vi "GetPosRef.vi"(0 "Entrée Variables d'Axes":T1={"OrdreBloc"="ni.var.psp://localhost/OPC/OPC1/esbimETH_1/module1/2AXBOC/E0_Ordre/Axe1_OrdreBloc", "Ordre UC"="ni.var.psp://localhost/OPC/OPC1/esbimETH_1/module1/2AXBOC/E0_Ordre/Axe1_OrdreUC", "CoteAAtteindre"="ni.var.psp://localhost/OPC/OPC1/esbimETH_1/module1/2AXBOC/E1_Position1/CoteAAtteindre", "Vitesse"="ni.var.psp://localhost/OPC/OPC1/esbimETH_1/module1/2AXBOC/E1_Position1/Vitesse", "Position codeur en pas"="ni.var.psp://localhost/OPC/OPC1/esbimETH_1/module1/2AXBOC/L4_PositionPas/Axe1_PositionCodeurEnPas", "Position Théorique"="ni.var.psp://localhost/OPC/OPC1/esbimETH_1/module1/2AXBOC/L0_Position/Axe1_PositionTheorique", "Message"="ni.var.psp://localhost/OPC/OPC1/esbimETH_1/module1/2AXBOC/L0_Position/Axe1_Messages", "Ecrire"="ni.var.psp://localhost/OPC/OPC1/esbimETH_1/module1/2AXBOC/ecrire", "Zone à écrire"="ni.var.psp://localhost/OPC/OPC1/esbimETH_1/module1/2AXBOC/zones_a_ecrire", "Numéro paramètre"="ni.var.psp://localhost/OPC/OPC1/esbimETH_1/module1/2AXBOC/E3_Parametres/NumeroParametre", "Ordre"="ni.var.psp://localhost/OPC/OPC1/esbimETH_1/module1/2AXBOC/E3_Parametres/Ordre", "Valeur"="ni.var.psp://localhost/OPC/OPC1/esbimETH_1/module1/2AXBOC/E3_Parametres/Valeur", "Valeur Lecture"="ni.var.psp://localhost/OPC/OPC1/esbimETH_1/module1/2AXBOC/L2_Parametres/Valeur", "Numéro paramètre Lecture"="ni.var.psp://localhost/OPC/OPC1/esbimETH_1/module1/2AXBOC/L2_Parametres/Numero", "Acquittement Lecture Ecriture"="", "Zone à Ecrire Pour Axe "=0, "Acquittement Ordre UC"=""}, 3 "error in (no error)":errorcluster caption="entrée d'erreur (pas d'erreur)") -> (9 "Références":i32[](array[numeric]), 10 "error out":errorcluster caption="sortie d'erreur")   [LabVIEW 2013]
uses:
  Controls/AdressesVariablesPartagees.ctl
  <vilib>/regexp/Match Regular Expression.xnode
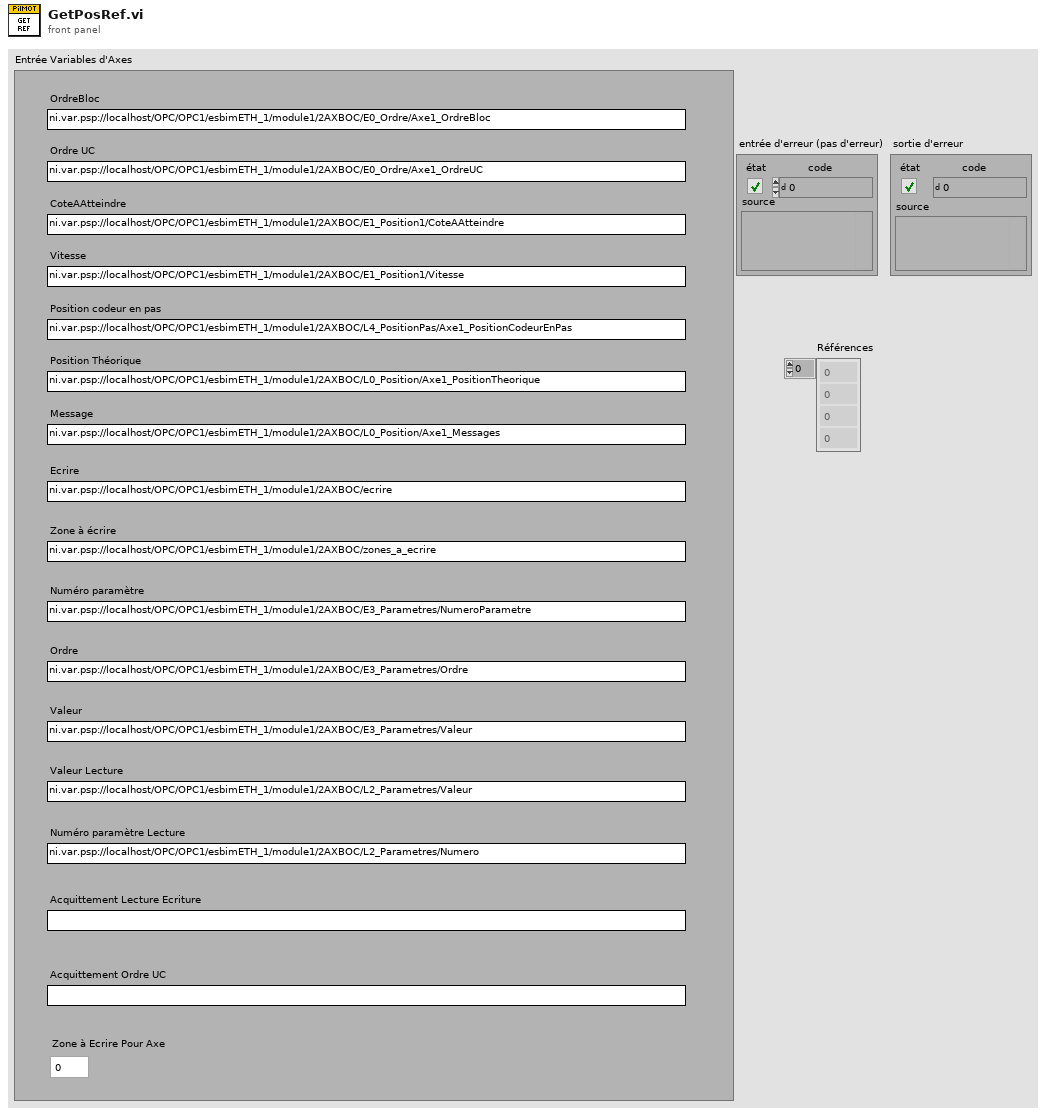
[diagram p1: front panel]
types:
  T1 = typedef "AdressesVariablesPartagees.ctl" = cluster{"OrdreBloc":string, "Ordre UC":string, "CoteAAtteindre":string, "Vitesse":string, "Position codeur en pas":string, "Position Théorique":string, "Message":string, "Ecrire":string, "Zone à écrire":string, "Numéro paramètre":string, "Ordre":string, "Valeur":string, "Valeur Lecture":string, "Numéro paramètre Lecture":string, "Acquittement Lecture Ecriture":string, "Zone à Ecrire Pour Axe ":u16, "Acquittement Ordre UC":string}
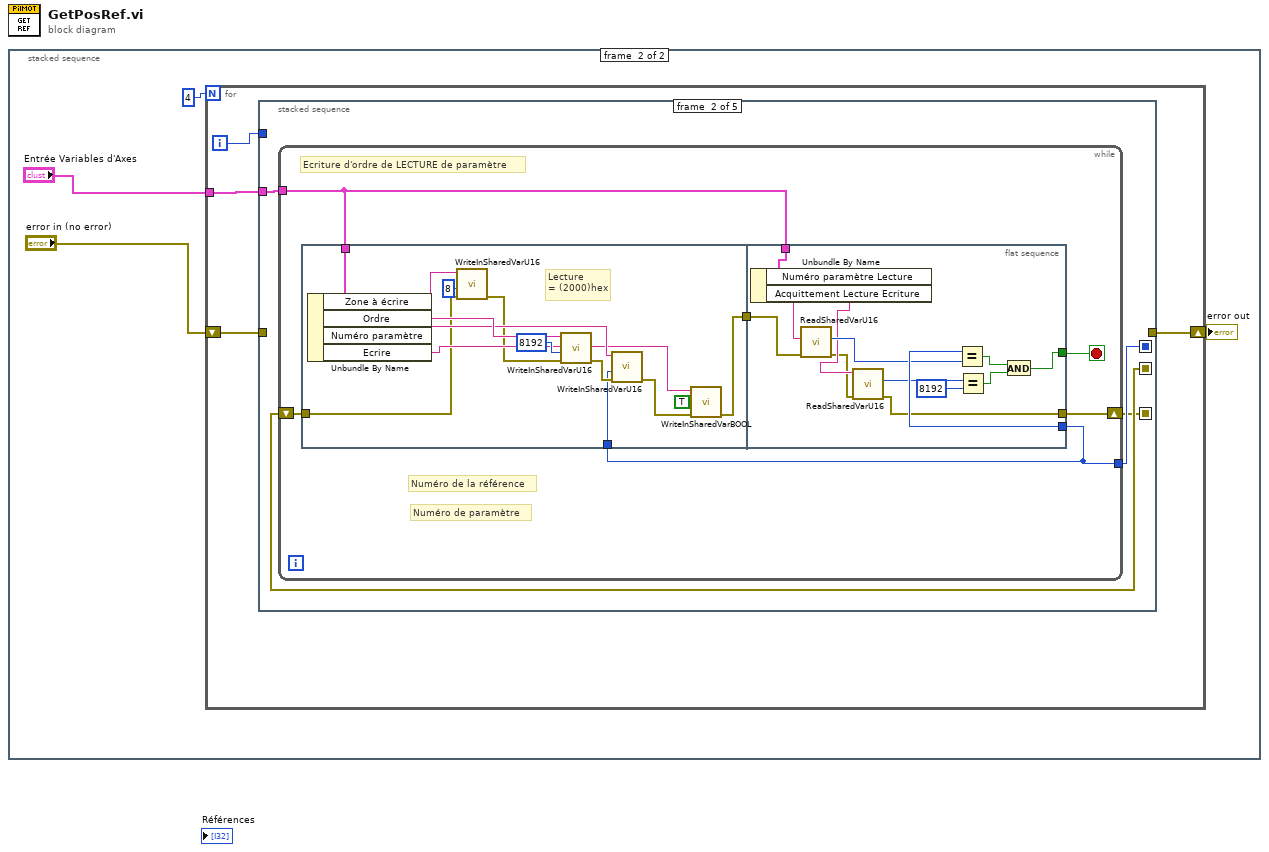
[diagram p0: block diagram]
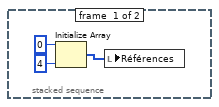
[diagram p2: hidden frame]
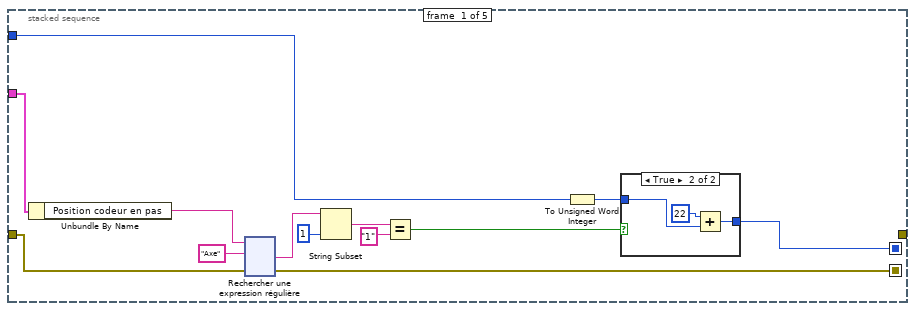
[diagram p3: hidden frame]
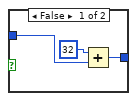
[diagram p4: hidden frame]
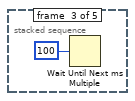
[diagram p5: hidden frame]
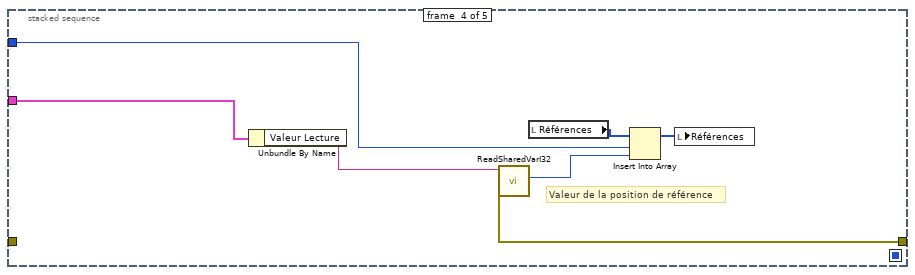
[diagram p6: hidden frame]
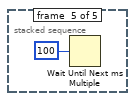
[diagram p7: hidden frame]
diagram:
  n1 = stacked-sequence {
    frame #0 {
      n2 = Initialize Array(0 ("élément"), 4 ("taille de la dimension")) -> (w1:i32[])
      n3 = local write "Références"(w1) -> ()
    }
    frame #1 {
      n4 = for {
        N: 4 -> [_]
        tunnel: "Entrée Variables d'Axes" -> [w11]
        shift-right: [w8] -> w5
        shift-left: "error in (no error)" -> [w9]
        i -> [w10]
        n5 = stacked-sequence {
          seq-local: [w16 _ _ _ _] -> [_ w146 _ _ _]
          seq-local: [w15 _ _ _ _] -> [_ w147 _ _ _]
          seq-local: [_ w145 _ _ _] -> [_ _ _ _ _]
          tunnel: w11 -> [w24 w148 _ w188 _]
          tunnel: w10 -> [w14 _ _ w186 _]
          tunnel: w9 -> [w12 _ _ _ _]
          tunnel: [_ _ _ w189 _] -> w8
          frame #0 {
            n6 = Unbundle By Name(w24) -> ("Position codeur en pas"=w17:string)
            n7 = xnode "Rechercher une expression régulière"("chaîne en entrée"=w17, "expression régulière"="Axe", "entrée d'erreur"=w12) -> ("après la correspondance"=w22:string, "sortie d'erreur"=w16:errorcluster)  [unwired: 3 in, 3 out]
            n8 = String Subset(string=w22, length (rest)=1 ("longueur (reste)")) -> (substring=w19:string)  [unwired: 1 in]
            n9 = Equal?(x=w19, y="1") -> (x = y?=w18:bool)
            n10 = To Unsigned Word Integer(number=w14) -> (unsigned 16bit integer=w13:u16)
            n11 = case shown="True" w18 {
              tunnel: w13 -> [w26 w29]
              tunnel: [w25 w28] -> w15
              frame False {
                n12 = Add(x=u16 32 ("Offset Paramètre"), y=w26) -> (x+y=w25:u16)
              }
              frame True {
                n13 = Add(x=u16 22 ("Offset Paramètre"), y=w29) -> (x+y=w28:u16)
              }
            }
          }
          frame #1 {
            n14 = while {
              tunnel: w148 -> [w151]
              tunnel: w147 -> [w153]
              shift-right: [w150] -> w145
              shift-left: w146 -> [w149]
              stop <- w152 stop-if-true
              # "Numéro de la référence"
              # "Ecriture d'ordre de LECTURE de paramètre"
              # "Numéro de paramètre"
              n15 = flat-sequence {
                tunnel: w151 -> [w168]
                tunnel: [w161] -> w154
                tunnel: w153 -> [w156]
                tunnel: w149 -> [w155]
                tunnel: [w172] -> w150
                tunnel: w154 -> [w178]
                tunnel: w153 -> [w181]
                tunnel: [w169] -> w152
                tunnel: w151 -> [w180]
                frame #0 {
                  # "Lecture \n= (2000)hex"
                  n16 = Unbundle By Name(w168) -> ("Zone à écrire"=w160:string, "Ordre"=w167:string, "Numéro paramètre"=w165:string, "Ecrire"=w163:string)
                  n17 = call "WriteInSharedVarU16.vi"("entrée d'erreur (pas d'erreur)"=w155, "données en entrée"=u16 8, "refnum de variable partagée en entrée"=w160) -> ("sortie d'erreur"=w158:errorcluster)  [unwired: 8 in]
                  n18 = call "WriteInSharedVarU16.vi"("entrée d'erreur (pas d'erreur)"=w158, "données en entrée"=u16 8192, "refnum de variable partagée en entrée"=w167) -> ("sortie d'erreur"=w164:errorcluster)  [unwired: 8 in]
                  n19 = call "WriteInSharedVarU16.vi"("entrée d'erreur (pas d'erreur)"=w164, "données en entrée"=w156, "refnum de variable partagée en entrée"=w165) -> ("sortie d'erreur"=w162:errorcluster)  [unwired: 8 in]
                  n20 = call "WriteInSharedVarBOOL.vi"("entrée d'erreur (pas d'erreur)"=w162, "données en entrée"=TRUE, "refnum de variable partagée en entrée"=w163) -> ("sortie d'erreur"=w161:errorcluster)  [unwired: 8 in]
                }
                frame #1 {
                  n21 = Unbundle By Name(w180) -> ("Numéro paramètre Lecture"=w179:string, "Acquittement Lecture Ecriture"=w176:string)
                  n22 = call "ReadSharedVarU16.vi"("entrée d'erreur (pas d'erreur)"=w178, "refnum de variable partagée en entrée"=w179) -> ("sortie d'erreur"=w173:errorcluster, "données en sortie"=w177:u16)  [unwired: 8 in]
                  n23 = call "ReadSharedVarU16.vi"("entrée d'erreur (pas d'erreur)"=w173, "refnum de variable partagée en entrée"=w176) -> ("sortie d'erreur"=w172:errorcluster, "données en sortie"=w175:u16)  [unwired: 8 in]
                  n24 = Equal?(x=w181, y=w177) -> (x = y?=w171:bool)
                  n25 = Equal?(x=w175, y=u16 8192) -> (x = y?=w170:bool)
                  n26 = And(x=w171, y=w170) -> (x .and. y?=w169:bool)
                }
              }
            }
          }
          frame #2 {
            n27 = Wait Until Next ms Multiple(millisecond multiple=u32 100 ("n millisecondes")) -> ()  [unwired: 1 out]
          }
          frame #3 {
            # "Valeur de la position de référence"
            n28 = Unbundle By Name(w188) -> ("Valeur Lecture"=w187:string)
            n29 = call "ReadSharedVarI32.vi"("refnum de variable partagée en entrée"=w187) -> ("sortie d'erreur"=w189:errorcluster, "données en sortie"=w185:i32)  [unwired: 9 in]
            n30 = local read "Références"() -> (w184:i32[])
            n31 = Insert Into Array(array=w184, index=w186, new element=w185) -> (w183:i32[])
            n32 = local write "Références"(w183) -> ()
          }
          frame #4 {
            n33 = Wait Until Next ms Multiple(millisecond multiple=u32 100 ("n millisecondes")) -> ()  [unwired: 1 out]
          }
        }
      }
      "error out" <- w5
    }
  }
